vi "test Find Disabled Custom Device.vi"(8 "error in":errorcluster, 11 "TestCase in":refnum<class "Scripting.lvclass">) -> (0 "error out":errorcluster, 3 "TestCase out":refnum<class "Scripting.lvclass">)   [LabVIEW 2020, in "Scripting.lvclass"]
uses:
  Scripting.lvclass
  <vilib>/addons/_JKI Toolkits/VI Tester/TestCase.llb/TestCase.lvclass
  Scripting/AIM MIL-STD-1553 Scripting.lvlib
  C:/dev/git/niveristand-custom-device-testing-tools/VeriStandScriptingTestCase/VeriStandScriptingTestCase.lvclass
  C:/Program Files (x86)/National Instruments/LabVIEW 2020/vi.lib/addons/_JKI Toolkits/VI Tester/TestCase.llb/TestCase.lvclass
  C:/dev/git/niveristand-aim-milStd1553-custom-device/Source/Custom Device Support/Tests/Unit/Scripting/Scripting.lvclass
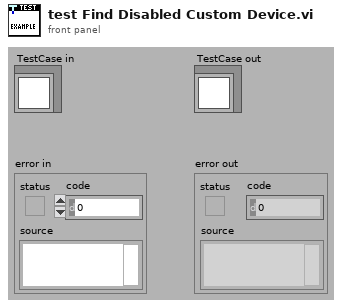
[diagram p1: front panel]
types:
  T1 = typedef "Custom Device API.lvlib/Custom Device Item Ref.ctl" = u64
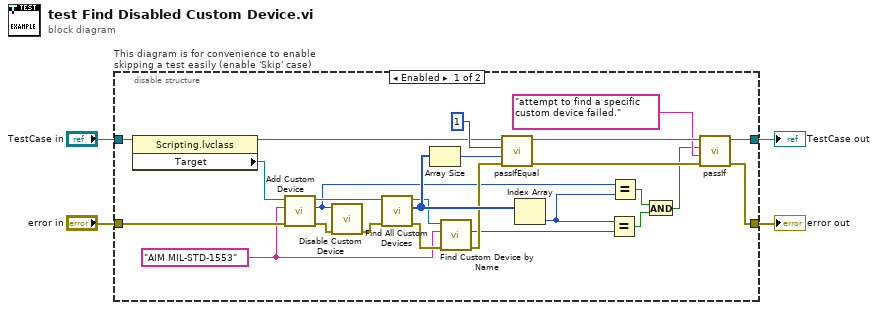
[diagram p0: block diagram]
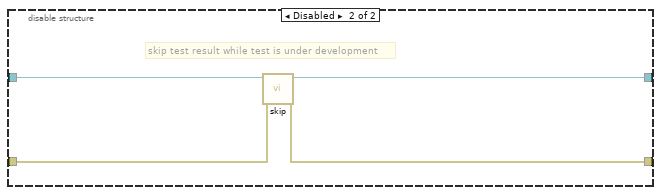
[diagram p2: hidden frame]
diagram:
  n1 = disable-structure "This diagram is for convenience to enable skipping a test easily (enable 'Skip' case)" shown="Enabled" {
    disable-tunnel: "TestCase in" -> [w23 w33]
    disable-tunnel: [w24 w31] -> w1
    disable-tunnel: [w25 w32] -> w3
    disable-tunnel: "error in" -> [w20 w30]
    frame Enabled {
      w5 = "AIM MIL-STD-1553" ("name")
      n2 = property class="Scripting.lvclass"(reference=w23) -> (reference out=w19:refnum<class "Scripting.lvclass">, "Target"=w21:refnum<k24>)  [unwired: 1 in, 1 out]
      n3 = call "Add Custom Device.vi"("error in"=w20, "custom device name"=w5, "target"=w21) -> ("error out"=w18:errorcluster, "custom device"=w10:T1, "target out"=w16:refnum<k24>)  [unwired: 6 in]
      n4 = call "Disable Custom Device.vi"("error in"=w18, "custom device ref"=w10) -> ("error out"=w17:errorcluster)  [unwired: 8 in, 1 out]
      n5 = call "Find All Custom Devices.vi"("error in"=w17, "target"=w16) -> ("error out"=w13:errorcluster, "custom devices"=w15:T1[], "target out"=w14:refnum<k24>)  [unwired: 7 in]
      n6 = Array Size(array=w15) -> (size(s)=w28:i32)
      n7 = call "Find Custom Device by Name.vi"("error in"=w13, "custom device name"=w5, "target"=w14) -> ("error out"=w12:errorcluster, "custom device"=w11:T1)  [unwired: 5 in, 2 out]
      n8 = call-dynamic "passIfEqual.vi"("error in (no error)"=w12, "y"=w28, "x"=1 ("disabled custom device"), "TestCase in"=w19) -> ("error out"=w27:errorcluster, "TestCase out"=w26:refnum<class "Scripting.lvclass">)  [unwired: 6 in]
      n9 = Index Array(array=w15) -> (element=w9:T1)  [unwired: 1 in]
      n10 = Equal?(x=w9, y=w11) -> (x = y?=w8:bool)
      n11 = Equal?(x=w10, y=w9) -> (x = y?=w7:bool)
      n12 = And(x=w7, y=w8) -> (x .and. y?=w6:bool)
      n13 = call-dynamic "passIf.vi"("error in (no error)"=w27, "message (\"\")"="attempt to find a specific custom device failed." ("message (\"\")"), "pass"=w6, "TestCase in"=w26) -> ("error out"=w25:errorcluster, "TestCase out"=w24:refnum<class "Scripting.lvclass">)  [unwired: 6 in]
    }
    frame Disabled {
      # "skip test result while test is under development"
      n14 = call <vilib>:"skip.vi"("error in (no error)"=w30, "TestCase in"=w33) -> ("error out"=w32:errorcluster, "TestCase out"=w31:refnum<class "Scripting.lvclass">)  [unwired: 8 in]
    }
  }
  "error out" <- w3
  "TestCase out" <- w1
